vi "poly_control_ref_from_name_multi.vi"(8 "error in (no error)":errorcluster, 9 "control names":string[](array[string]), 10 "vi ref":refnum<vi>) -> (0 "error out":errorcluster, 1 "ctrl refs":refnum<vi>[](array[refnum]), 2 "vi ref dup":refnum<vi>, 4 "found?":bool[](array[boolean]))   [LabVIEW 2015, in "_ref_tools_polys.lvlib"]
uses:
  _ref_tools_polys.lvlib
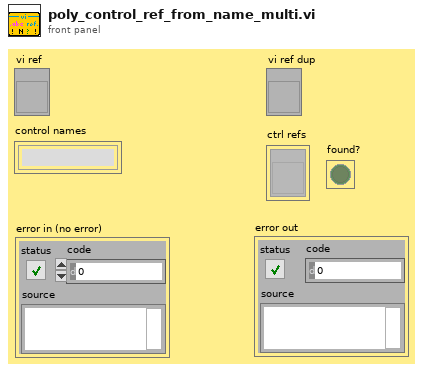
[diagram p1: front panel]
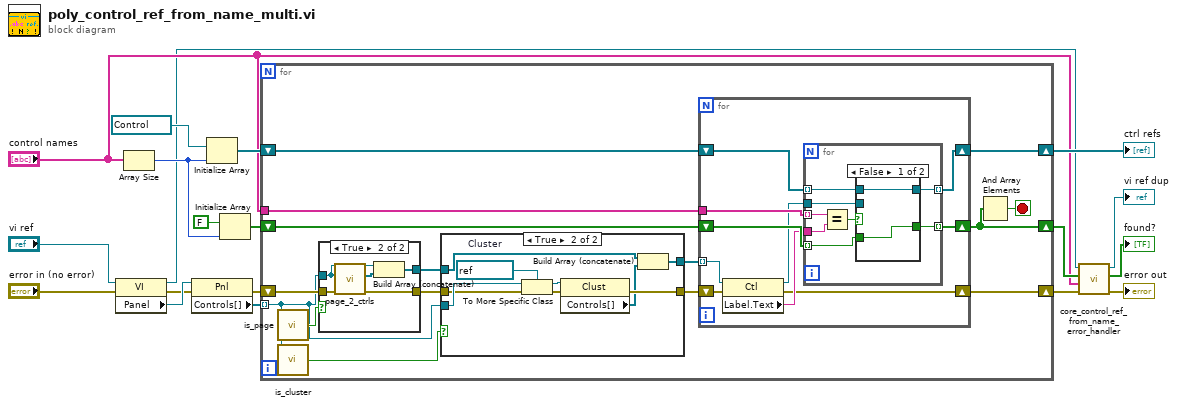
[diagram p0: block diagram]
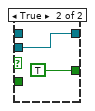
[diagram p3: hidden frame]
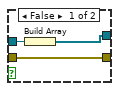
[diagram p4: hidden frame]
diagram:
  n1 = property class="VI"(reference="vi ref", error in="error in (no error)") -> (reference out=w2:refnum<vi>, error out=w10:errorcluster, "Panel"=w12:refnum<vi>)
  n2 = Array Size(array="control names") -> (size(s)=w15:i32)
  n3 = property class="Pnl"(reference=w12, error in=w10) -> (error out=w9:errorcluster, "Controls[]"=w11:refnum<vi>[])  [unwired: 1 out]
  n4 = Initialize Array(refnum<vi> refnum ("ctrl ref"), w15) -> (w16:refnum<vi>[])
  n5 = Initialize Array(FALSE, w15) -> (w13:bool[])
  n6 = for {
    tunnel: w11 -> [w24] mode=indexing
    tunnel: "control names" -> [w34]
    shift-right: [w28] -> w7
    shift-left: w13 -> [w32]
    shift-right: [w29] -> w8
    shift-left: w16 -> [w33]
    shift-right: [w26] -> w5
    shift-left: w9 -> [w30]
    stop <- w27 stop-if-true
    n7 = call "is_page.vi"("ctrl ref"=w24) -> ("is page?"=w31:bool)
    n8 = call "is_cluster.vi"("ctrl ref"=w24) -> ("is page?"=w25:bool)
    n9 = case shown="True" w31 {
      tunnel: w24 -> [w70 w73]
      tunnel: [w69 w72] -> w20
      tunnel: w30 -> [w68 w75]
      tunnel: [w68 w71] -> w23
      frame False {
        n10 = Build Array(w70) -> (w69:refnum<vi>[])
      }
      frame True {
        n11 = call "page_2_ctrls.vi"("Error in"=w75, "ctrl ref"=w73) -> ("Error out"=w71:errorcluster, "ctrls in pages"=w74:refnum<vi>[])  [unwired: 3 in, 1 out]
        n12 = Build Array (concatenate)(w73, w74) -> (w72:refnum<vi>[])
      }
    }
    n13 = case shown="True" w25 {
      tunnel: w24 -> [_ w44]
      tunnel: w23 -> [w35 w43]
      tunnel: [w35 w41] -> w22
      tunnel: [w36 w37] -> w21
      tunnel: w20 -> [w36 w39]
      frame False {
      }
      frame True {
        w45 = refnum<vi> refnum  # Cluster
        n14 = To More Specific Class(target class=w45, reference=w44, error in=w43) -> (specific class reference=w40:refnum<vi>, error out=w42:errorcluster)
        n15 = property class="Clust"(reference=w40, error in=w42) -> (error out=w41:errorcluster, "Controls[]"=w38:refnum<vi>[])  [unwired: 1 out]
        n16 = Build Array (concatenate)(w39, w38) -> (w37:refnum<vi>[])
      }
    }
    n17 = for {
      tunnel: w34 -> [w55]
      tunnel: w21 -> [w50] mode=indexing
      shift-right: [w46] -> w26
      shift-left: w22 -> [w49]
      shift-right: [w51] -> w29
      shift-left: w33 -> [w54]
      shift-right: [w52] -> w28
      shift-left: w32 -> [w53]
      n18 = property class="Ctl"(reference=w50, error in=w49) -> (reference out=w47:refnum<vi>, error out=w46:errorcluster, "Label.Text"=w48:string)
      n19 = for {
        tunnel: w55 -> [w63] mode=indexing
        tunnel: w53 -> [w59] mode=indexing
        tunnel: w54 -> [w62] mode=indexing
        tunnel: [w61] -> w51 mode=indexing
        tunnel: [w58] -> w52 mode=indexing
        tunnel: w48 -> [w57]
        tunnel: w47 -> [w56]
        n20 = Equal?(x=w63, y=w57) -> (x = y?=w60:bool)
        n21 = case shown="False" w60 {
          tunnel: w62 -> [w65 _]
          tunnel: [w65 w66] -> w61
          tunnel: w59 -> [w64 _]
          tunnel: [w64 TRUE] -> w58
          tunnel: w56 -> [_ w66]
          frame False {
          }
          frame True {
          }
        }
      }
    }
    n22 = And Array Elements(Boolean array=w28) -> (logical AND=w27:bool)
  }
  "ctrl refs" <- w8
  n23 = call "core_control_ref_from_name_error_handler.vi"("error in"=w5, "control names"="control names", "found?"=w7, "vi ref"=w2) -> ("error out"=→"error out":errorcluster, "found? duplicate"=→"found?":bool[], "vi ref dup"=→"vi ref dup":refnum<vi>)  [unwired: 5 in]
